vi "DSF.Engine.Runtime.Plugin.Get Interface.vi"(8 "error in (no error)":errorcluster, 11 "Plugin Runtime in":refnum<class "DSF.Engine.Runtime.Plugin.lvclass">) -> (0 "error out":errorcluster, 2 "Plugin Interface":refnum<class "DSF.Engine.Interface.Plugin.lvclass">, 3 "Plugin Runtime out":refnum<class "DSF.Engine.Runtime.Plugin.lvclass">)   [LabVIEW 2016, in "DSF.Engine.lvlib" / "DSF.Engine.Runtime.Plugin.lvclass"]
uses:
  DSF.Engine.Runtime.Plugin.lvclass
  Interface/DSF.Engine.Interface.Plugin.lvclass
  DSF.Engine.Runtime.Plugin.lvclass/DSF.Engine.Runtime.Plugin.ctl
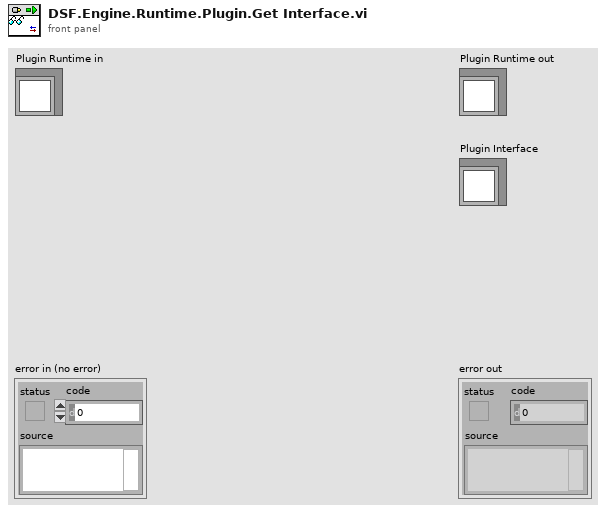
[diagram p1: front panel]
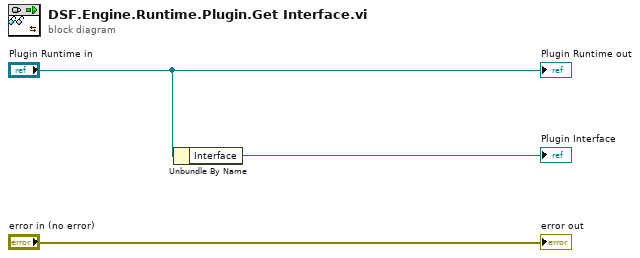
[diagram p0: block diagram]
diagram:
  n1 = Unbundle By Name("Plugin Runtime in") -> ("Interface"=→"Plugin Interface":refnum<class "DSF.Engine.Interface.Plugin.lvclass">)
  "error out" <- "error in (no error)"
  "Plugin Runtime out" <- "Plugin Runtime in"
